vi "remove_array_outliers 11-16-2017.vi"(7 "n standard devs to filter":dbl=0.0001 min=0.0001 max=10000.0 format="%0.2f", 10 "input array":dbl[](array[numeric])) -> (2 "filtered array out":dbl[](array[numeric]))   [LabVIEW 2014]
uses:
  <vilib>/Analysis/NI_AALBase.lvlib
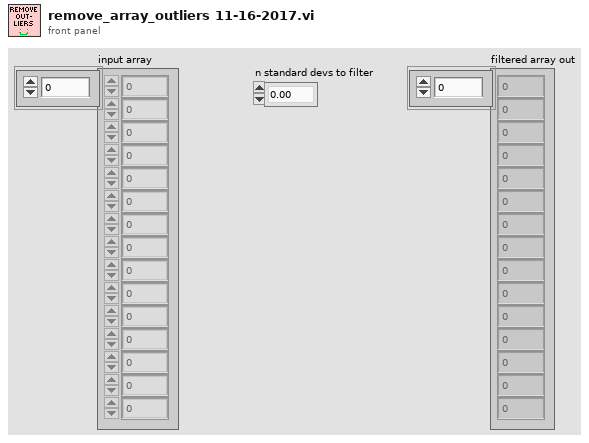
[diagram p1: front panel]
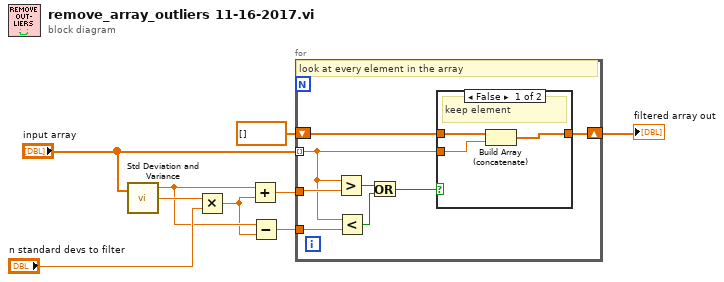
[diagram p0: block diagram]
diagram:
  n1 = call <vilib>:"Std Deviation and Variance.vi"("X"="input array") -> ("mean"=w7:dbl, "standard deviation"=w9:dbl)  [unwired: 1 in, 1 out]
  n2 = Multiply(x=w9, y="n standard devs to filter") -> (x*y=w6:dbl)
  n3 = Add(x=w7, y=w6) -> (x+y=w4:dbl)
  n4 = Subtract(x=w7, y=w6) -> (x-y=w3:dbl)
  n5 = for {
    tunnel: "input array" -> [w12] mode=indexing
    tunnel: w4 -> [w17]
    tunnel: w3 -> [w15]
    shift-right: [w11] -> w1
    shift-left: dbl[] [] -> [w10]
    # "look at every element in the array"
    n6 = Greater?(x=w12, y=w17) -> (0:w16:bool)
    n7 = Less?(x=w12, y=w15) -> (x < y?=w14:bool)
    n8 = Or(x=w16, y=w14) -> (x .or. y?=w13:bool)
    n9 = case shown="False" w13 {
      tunnel: w12 -> [w20 _]
      tunnel: [w19 w21] -> w11
      tunnel: w10 -> [w18 w21]
      frame False {
        # "keep element"
        n10 = Build Array (concatenate)(w18, w20) -> (w19:dbl[])
      }
      frame True {
        # "discard element"
      }
    }
  }
  "filtered array out" <- w1
